vi "Read Raw.vi"(8 "error in (no error)":errorcluster, 11 "senseHatDisplay in":refnum<class "RPI.SenseHat.Display.lvclass">) -> (0 "error out":errorcluster, 2 "Data":u8[](array[numeric]), 3 "senseHatDisplay out":refnum<class "RPI.SenseHat.Display.lvclass">)   [LabVIEW 2020, in "RPI.SenseHat.Display.lvlib" / "RPI.SenseHat.Display.lvclass"]
doc: "Reads the raw data of the physical display. Will return 192 bytes.\nThe layout of the LED buffer:\n Row 1: R R R R R R R R G G G G G G G G B B B B B B B B\n Row 2: R R R R R R R R G G G G G G G G B B B B B B B B\n ...\n Row 8: R R R R R R R R G G G G G G G G B B B B B B B B\n\nNote: Each color component is only 5 bits long, i.e. 0=darkest and 31=brightest."
uses:
  RPI.SenseHat.Display.lvclass
  RPI.SenseHat.Display.lvclass/RPI.SenseHat.Display.ctl
  RPI/Classes/mainI2CDevice/mainI2CDevice.lvclass
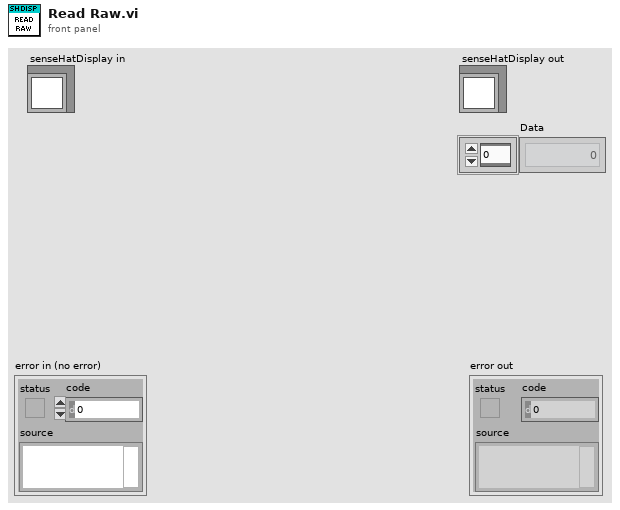
[diagram p1: front panel]
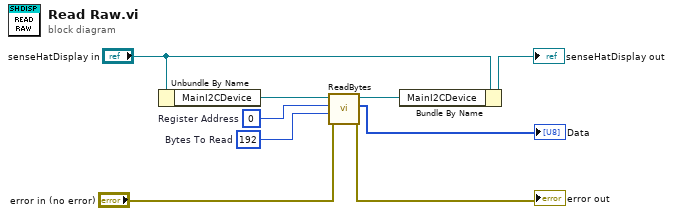
[diagram p0: block diagram]
diagram:
  w1 = u8 0  # Register Address
  w2 = u8 192  # Bytes To Read
  n1 = Unbundle By Name("senseHatDisplay in") -> ("MainI2CDevice"=w5:refnum<class "mainI2CDevice.lvclass">)
  n2 = call "ReadBytes.vi"("error in (no error)"="error in (no error)", "Bytes To Read"=w2, "Register Address"=w1, "mainI2CDevice in"=w5) -> ("error out"=→"error out":errorcluster, "Data"=→"Data":u8[], "mainI2CDevice out"=w4:refnum<class "mainI2CDevice.lvclass">)  [unwired: 5 in]
  n3 = Bundle By Name(cluster="senseHatDisplay in", "MainI2CDevice"=w4) -> (→"senseHatDisplay out":refnum<class "RPI.SenseHat.Display.lvclass">)
